vi "Retry State on Error.vi"(4 "milliseconds to wait (500 ms)":u32=500, 5 "Error Code":i32(ring) items=["No error", "Argument error", "Memory is full", "Out of zone", "End of file", "File already open", "Generic file I/O error", "File not found", "File permission error", "Disk is full", "Duplicate path", "Too many files open", "System feature not enabled", "Resource file not found", "Cannot add resource", "Resource not found", "Image not found", "Image memory error", "Pen does not exist", "Config type invalid", "Config token not found", "Config parse error", "Config memory error", "Bad external code format", "Bad external code offset", "External code not present", "Null window", "Destroy window error", "Null menu", "Print aborted", "Bad print record", "Print driver error", "Windows error during printing", "Memory error during printing", "Print dialog error", "Generic print error", "Invalid device refnum", "Device not found", "Device parameter error", "Device unit error", "Cannot open device", "Device call aborted", "Generic error", "Cancelled by user", "Object ID too low", "Object ID too high", "Object not in heap", "Unknown heap", "Unknown object (invalid DefProc)", "Unknown object (DefProc not in table)", "Message out of range", "Invalid (null) method", "Unknown message", "Manager call not supported", "Bad address", "Network operation in progress", "Network operation timed out", "Connection is busy", "Network attribute not supported", "Network error", "Address in use", "System out of memory", "Connection aborted", "Connection refused", "Not connected", "Already connected", "Connection closed", "Initialization error (interapplication manager)", "Bad occurrence", "Wait on unbound occurrence handler", "Occurrence queue overflow", "Datalog type conflict", "Unused", "Unrecognized type (interapplication manager)", "Memory corrupt", "Failed to make temporary DLL", "Old CIN version", "Drag socket not found", "Failed to load drop-object", "Failed to register OLE object", "Failed to release OLE object", "Format specifier type mismatch", "Unknown format specifier", "Too few format specifiers", "Too many format specifiers", "Scan failed", "Newer CIN version", "OLE Convert", "Runtime menu error", "Password tampered", "Unknown error code"], 6 "Opposite End (f)":bool, 7 "State":string, 8 "error in (no error)":errorcluster, 9 "timeout in ms (-1)":i32, 10 "Parameters":string, 11 "queue in":refnum<queue>) -> (0 "error out":errorcluster, 1 "timed out?":bool, 2 "Detected?":bool, 3 "queue out":refnum<queue>)   [LabVIEW 2011]
doc: "Enqueues a single element to the state machine. Inputs are State and Parameters to facilitate coding.\n\n\nVersion 1.0 - 10/21/2009\n\nPhaeron, Inc.\nwww.phaeron.com\ninfo@phaeron.com"
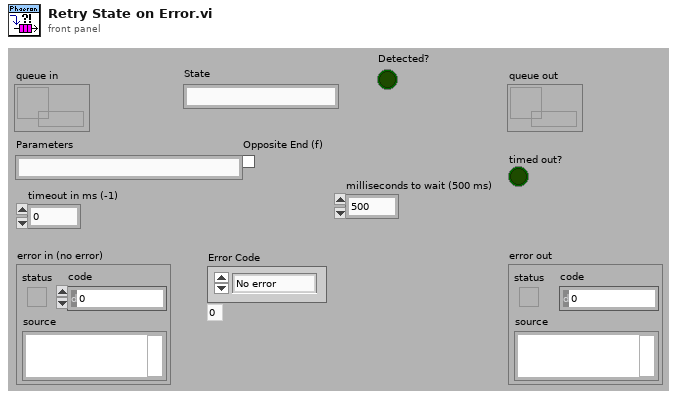
[diagram p1: front panel]
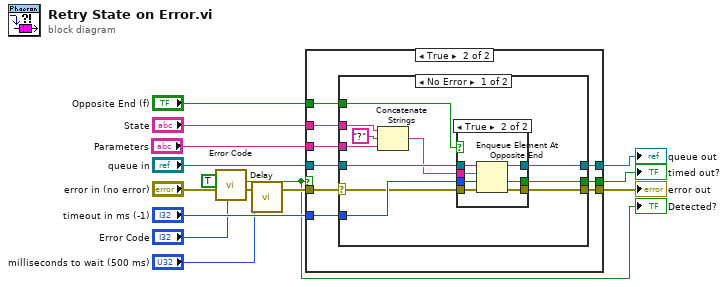
[diagram p0: block diagram]
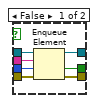
[diagram p3: hidden frame]
diagram:
  n1 = call "Error Code.vi"("Error Code"="Error Code", "error in (no error)"="error in (no error)", "Suppress? (T)"=TRUE ("Suppress? (F)")) -> ("error out"=w4:errorcluster, "Detected?"=w1:bool)  [unwired: 7 in]
  "Detected?" <- w1
  n2 = call "Delay.vi"("error in (no error)"=w4, "milliseconds to wait (1 ms)"="milliseconds to wait (500 ms)") -> ("error out"=w3:errorcluster)  [unwired: 17 in]
  n3 = case shown="True" w1 {
    tunnel: "Opposite End (f)" -> [_ w26]
    tunnel: [w16 w25] -> w14
    tunnel: [_ w24] -> w13
    tunnel: "timeout in ms (-1)" -> [_ w23]
    tunnel: "queue in" -> [w17 w22]
    tunnel: [w17 w21] -> w10
    tunnel: "State" -> [_ w20]
    tunnel: "Parameters" -> [_ w19]
    tunnel: w3 -> [w16 w18]
    frame False {
    }
    frame True {
      n4 = case shown="No Error" w18 {
        selector: w18 -> [w31 w53]
        tunnel: w26 -> [w27 _]
        tunnel: [w30 w53] -> w25
        tunnel: [w29 _] -> w24
        tunnel: w23 -> [w32 _]
        tunnel: w22 -> [w33 w52]
        tunnel: [w34 w52] -> w21
        tunnel: w20 -> [w37 _]
        tunnel: w19 -> [w36 _]
        frame No Error {
          n5 = Concatenate Strings(w37, "?" ("string"), w36) -> (w28:string)
          n6 = case shown="True" w27 {
            tunnel: w31 -> [w44 w50]
            tunnel: [w43 w51] -> w30
            tunnel: [w42 w45] -> w29
            tunnel: w32 -> [w41 w49]
            tunnel: w33 -> [w40 w47]
            tunnel: [w39 w46] -> w34
            tunnel: w28 -> [w38 w48]
            frame False {
              n7 = Enqueue Element(queue=w40, element=w38, timeout in ms (-1)=w41, error in (no error)=w44) -> (queue out=w39:refnum<queue>, timed out?=w42:bool, error out=w43:errorcluster)
            }
            frame True {
              n8 = Enqueue Element At Opposite End(queue=w47, element=w48, timeout in ms (-1)=w49, error in (no error)=w50) -> (queue out=w46:refnum<queue>, timed out?=w45:bool, error out=w51:errorcluster)
            }
          }
        }
        frame Error {
        }
      }
    }
  }
  "error out" <- w14
  "timed out?" <- w13
  "queue out" <- w10
